vi "Query Voltage Current Settings.vi"(7 "Slave Address":i32=-1 min=-1 max=30 step=1, 8 "error":errorcluster, 11 "VISA":refnum<visa-resource-name>) -> (0 "error out":errorcluster, 1 "Current Limit":dbl format="%.3f", 2 "Voltage Limit":dbl format="%.3f", 3 "VISA out":refnum<visa-resource-name>)   [LabVIEW 2025, in "TDK-Lambda GEN LAN Series.lvlib"]
doc: "Returns the voltage and current limit settings. \nThese settings may not be the same as the actual output voltage and current"
uses:
  <userlib>/TDK-Lambda GEN LAN Series/TDK-Lambda GEN LAN Series.lvlib
panel:
  # "TDK-Lambda Genesys \n LAN\n  DC Power Supplies"
  # "Read Voltage and \n Current Settings"
  # "Amps"
  # "Volts"
  # "(c) 2019 TDK-Lambda.  ALL RIGHTS RESERVED."
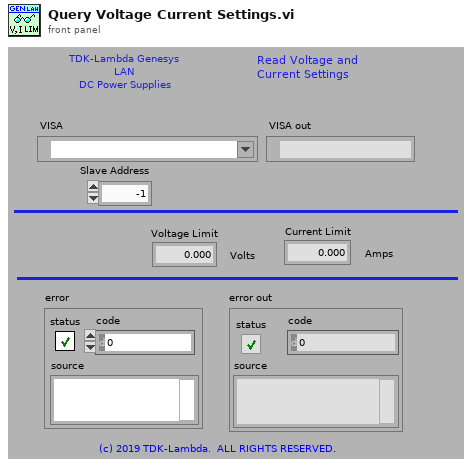
[diagram p1: front panel]
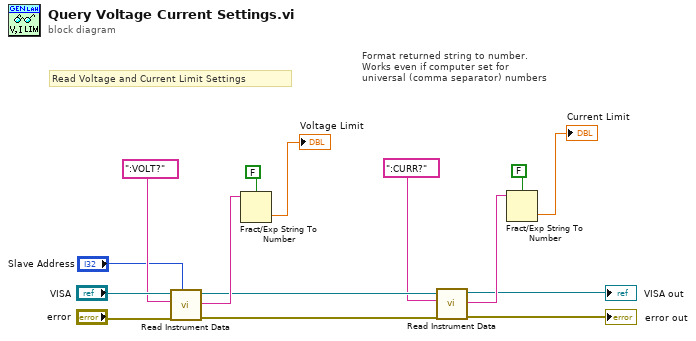
[diagram p0: block diagram]
diagram:
  # "Format returned string to number.\nWorks even if computer set for \nuniversal (comma separator) numbers"
  # "Read Voltage and Current Limit Settings"
  n1 = call <userlib>:"Read Instrument Data.vi"("Slave Address"="Slave Address", "error"="error", "Query"=":VOLT?", "VISA"="VISA") -> ("error out"=w7:errorcluster, "Response"=w11:string, "VISA out"=w8:refnum<visa-resource-name>)  [unwired: 4 in, 1 out]
  n2 = Fract/Exp String To Number(use system decimal point (T)=FALSE, string=w11) -> (number=→"Voltage Limit":dbl)  [unwired: 2 in, 1 out]
  n3 = call <userlib>:"Read Instrument Data.vi"("error"=w7, "Query"=":CURR?", "VISA"=w8) -> ("error out"=→"error out":errorcluster, "Response"=w10:string, "VISA out"=→"VISA out":refnum<visa-resource-name>)  [unwired: 5 in, 1 out]
  n4 = Fract/Exp String To Number(use system decimal point (T)=FALSE, string=w10) -> (number=→"Current Limit":dbl)  [unwired: 2 in, 1 out]
